vi "Measure.vi"(8 "error in (no error)":errorcluster, 9 "Measurement Type (Voltage)":string(combo)="MEAS:VOLT?", 11 "VISA resource name":refnum<visa-resource-name>) -> (0 "error out":errorcluster, 2 "Measurement":dbl format="%.2p", 3 "VISA resource name out":refnum<visa-resource-name>)   [LabVIEW 2012, in "Agilent E364X Series.lvlib"]
doc: "This VI takes a measurement on the output signal and returns the measured value."
uses:
  Agilent E364X Series.lvlib
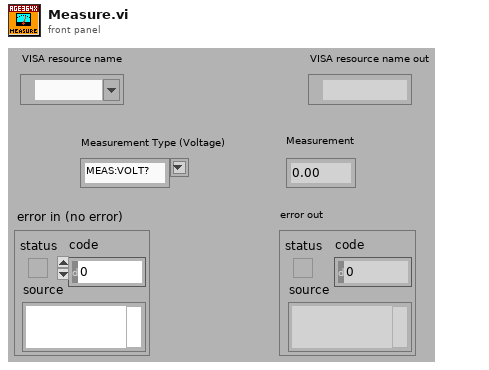
[diagram p1: front panel]
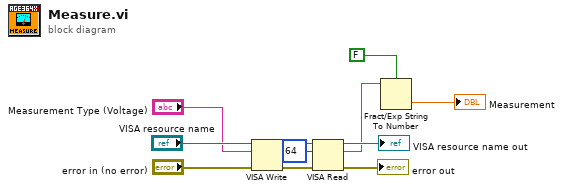
[diagram p0: block diagram]
diagram:
  n1 = VISA Write(VISA resource name="VISA resource name", write buffer="Measurement Type (Voltage)", error in (no error)="error in (no error)") -> (VISA resource name out=w3:refnum<visa-resource-name>, error out=w11:errorcluster)  [unwired: 1 out]
  n2 = VISA Read(VISA resource name=w3, byte count=u32 64, error in (no error)=w11) -> (VISA resource name out=→"VISA resource name out":refnum<visa-resource-name>, read buffer=w5:string, error out=→"error out":errorcluster)  [unwired: 1 out]
  n3 = Fract/Exp String To Number(use system decimal point (T)=FALSE, string=w5) -> (number=→"Measurement":dbl)  [unwired: 2 in, 1 out]
